vi "Pre-Install Custom Action.vi"(10 "Variant":variant) -> (0 "error out":errorcluster)   [LabVIEW 2014]
uses:
  RasPi Compiler/Compile and Download App/Custom Controls/Local Setup Parameters.ctl
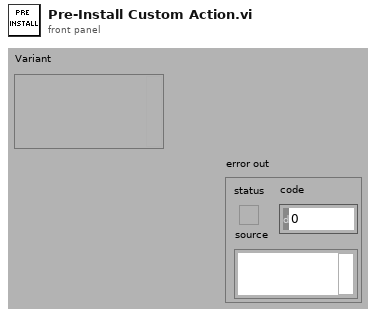
[diagram p1: front panel]
types:
  T1 = typedef "Local Setup Parameters.ctl" = enum16{"Add Last VI", "Read Last VI", "Add Board IP", "Remove Board IP", "Read All Board IP", "Add Runtime Version", "Read Runtime Version", "Add Package Version", "Read Package Version"}
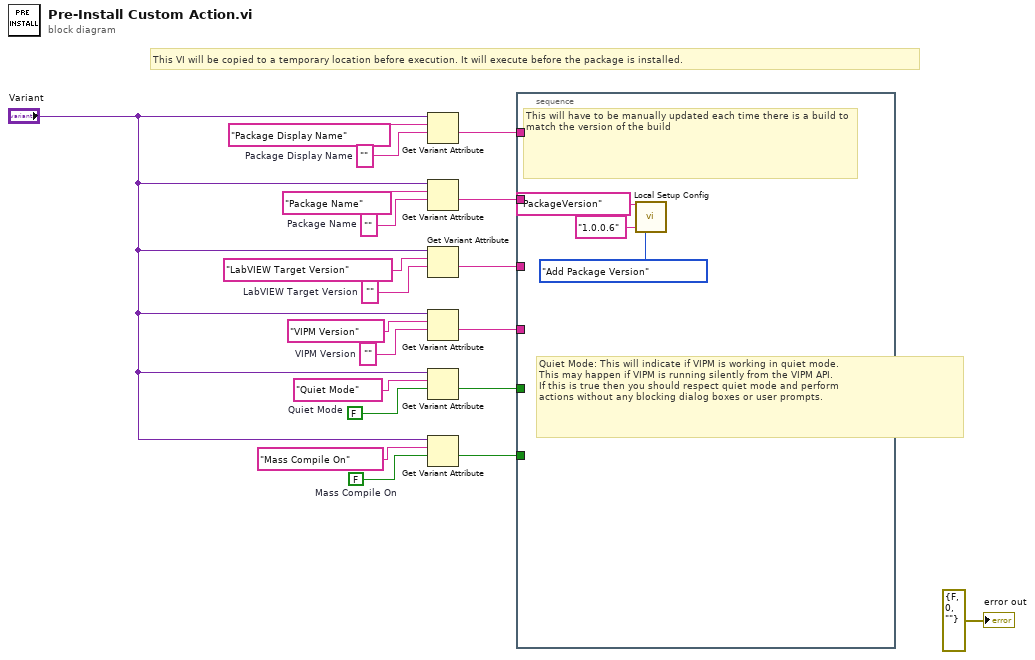
[diagram p0: block diagram]
diagram:
  w1 = FALSE  # Mass Compile On
  w3 = ""  # Package Display Name
  w10 = FALSE  # Quiet Mode
  w13 = ""  # VIPM Version
  w15 = ""  # LabVIEW Target Version
  w17 = ""  # Package Name
  # "This VI will be copied to a temporary location before execution. It will execute before the package is installed."
  n1 = Get Variant Attribute(Variant="Variant", name="Package Display Name", default value (empty Variant)=w3) -> (value=w9:string)  [unwired: 1 in, 3 out]
  n2 = Get Variant Attribute(Variant="Variant", name="Package Name", default value (empty Variant)=w17) -> (value=w8:string)  [unwired: 1 in, 3 out]
  n3 = Get Variant Attribute(Variant="Variant", name="LabVIEW Target Version", default value (empty Variant)=w15) -> (value=w7:string)  [unwired: 1 in, 3 out]
  n4 = Get Variant Attribute(Variant="Variant", name="VIPM Version", default value (empty Variant)=w13) -> (value=w6:string)  [unwired: 1 in, 3 out]
  n5 = Get Variant Attribute(Variant="Variant", name="Quiet Mode", default value (empty Variant)=w10) -> (value=w5:bool)  [unwired: 1 in, 3 out]
  n6 = Get Variant Attribute(Variant="Variant", name="Mass Compile On", default value (empty Variant)=w1) -> (value=w4:bool)  [unwired: 1 in, 3 out]
  n7 = stacked-sequence {
    tunnel: w9 -> [_]
    tunnel: w8 -> [_]
    tunnel: w7 -> [_]
    tunnel: w6 -> [_]
    tunnel: w5 -> [_]
    tunnel: w4 -> [_]
    frame #0 {
      # "Quiet Mode: This will indicate if VIPM is working in quiet mode.\nThis may happen if VIPM is running silently from the VIPM API.\nIf this is true then you should respect quiet mode and perform\nactions without any blocking dialog boxes or user prompts."
      # "This will have to be manually updated each time there is a build to match the version of the build"
      n8 = call "Local Setup Config.vi"("KeyName"="PackageVersion", "Local Setup Param"=Local_Setup_Parameters."Add Package Version", "KeyValue"="1.0.0.6") -> ()  [unwired: 9 in, 4 out]
    }
  }
  "error out" <- errorcluster {"status"=FALSE, "code"=0, "source"=""} ("error out")
